vi "ad get range info.vi"(7 "info":T1, 8 "error in (no error)":errorcluster, 9 "range":i32, 10 "cha":i32, 11 "adh":i32) -> (0 "error out":errorcluster, 3 "function return":i32, 5 "info out":T1)   [LabVIEW 2021, in "libad4.lvlib"]
doc: "LIBAD4 function: ad_get_range_info (int32_t adh, int32_t cha, int32_t range, struct ad_range_info *info);\n\nReturns information about the specified measurement range."
uses:
  <userlib>/libad4/libad4.lvlib
  <userlib>/libad4/controls/ad range info.ctl
  <userlib>/libad4/libad4.dll
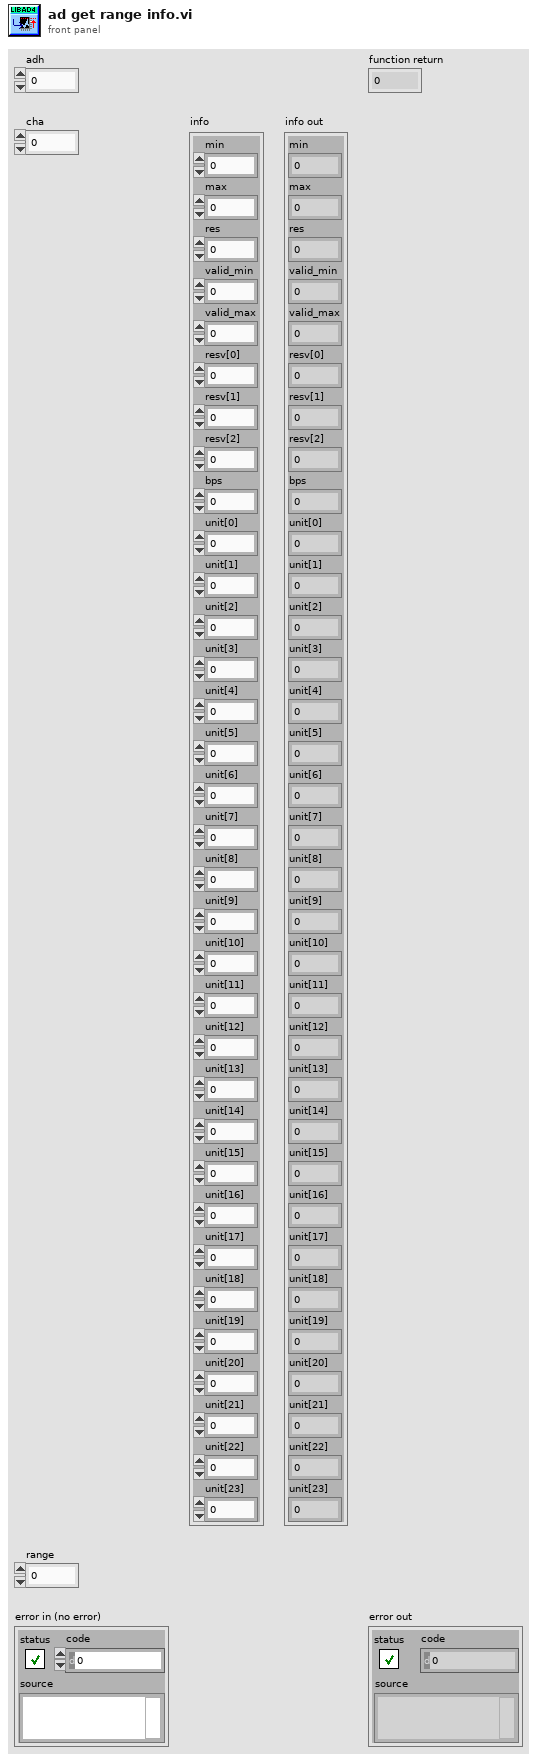
[diagram p1: front panel]
types:
  T1 = typedef "libad4.lvlib/ad range info.ctl" = cluster{"min":dbl, "max":dbl, "res":dbl, "valid_min":dbl, "valid_max":dbl, "resv[0]":dbl, "resv[1]":dbl, "resv[2]":dbl, "bps":i32, "unit[0]":i8, "unit[1]":i8, "unit[2]":i8, "unit[3]":i8, "unit[4]":i8, "unit[5]":i8, "unit[6]":i8, "unit[7]":i8, "unit[8]":i8, "unit[9]":i8, "unit[10]":i8, "unit[11]":i8, "unit[12]":i8, "unit[13]":i8, "unit[14]":i8, "unit[15]":i8, "unit[16]":i8, "unit[17]":i8, "unit[18]":i8, "unit[19]":i8, "unit[20]":i8, "unit[21]":i8, "unit[22]":i8, "unit[23]":i8}
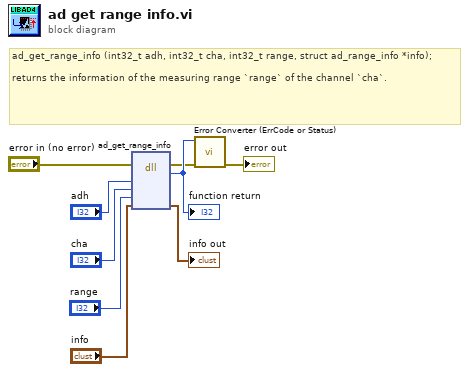
[diagram p0: block diagram]
diagram:
  # "ad_get_range_info (int32_t adh, int32_t cha, int32_t range, struct ad_range_info *info);\n\nreturns the information of the measuring range `range` of the channel `cha`."
  n1 = dll-call lib="C:/Program Files/National Instruments/LabVIEW 2021/user.lib/libad4/libad4.*" fn="ad_get_range_info"(error in="error in (no error)", "adh"="adh", "cha"="cha", "range"="range", "info"="info") -> (error out=w2:errorcluster, w9:i32, "info"=→"info out":T1)  [unwired: 5 in, 1 out]
  "function return" <- w9
  n2 = call <userlib>:"Error Converter (ErrCode or Status).vi"("error in (no error)"=w2, "error code"=w9) -> ("error out"=→"error out":errorcluster)  [unwired: 9 in]
